vi "Variant to Meta Data.vi"(8 "Error In":errorcluster, 9 "Name":string, 11 "Value":variant) -> (0 "Error Out":errorcluster, 1 "Name out":string, 2 "deleted path":path, 3 "Meta data":string)   [LabVIEW 2016]
uses:
  <vilib>/Utility/config.llb/NI_LVConfig.lvlib
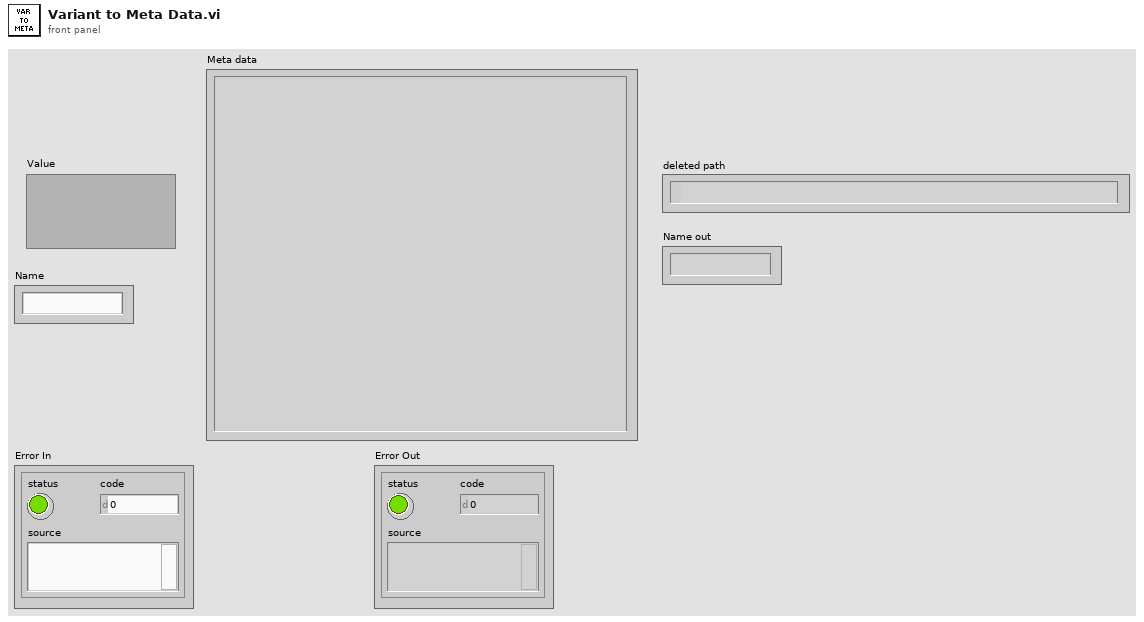
[diagram p1: front panel]
types:
  T1 = typedef "NI_LVConfig.lvlib/Config Data RefNum.ctl" = refnum<k1>
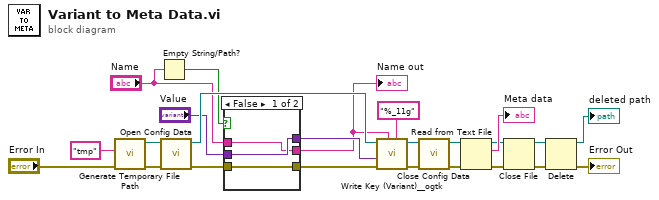
[diagram p0: block diagram]
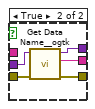
[diagram p2: hidden frame]
diagram:
  n1 = call <vilib>:"Generate Temporary File Path.vi"("error in (no error)"="Error In", "Temporary File Extension (tmp)"="tmp") -> ("error out"=w11:errorcluster, "Unique Temporary File Path"=w23:path)  [unwired: 8 in]
  n2 = Empty String/Path?(string/path="Name") -> (empty?=w7:bool)
  n3 = call <vilib>:"Open Config Data.vi"("error in (no error)"=w11, "configuration file path"=w23) -> ("error out"=w6:errorcluster, "refnum"=w22:T1)  [unwired: 7 in, 1 out]
  n4 = case shown="False" w7 {
    tunnel: "Value" -> [w27 w32]
    tunnel: [w25 w31] -> w2
    tunnel: w6 -> [w26 w30]
    tunnel: [w26 w29] -> w5
    tunnel: [w27 w28] -> w4
    tunnel: "Name" -> [w25 _]
    frame False {
    }
    frame True {
      n5 = call <userlib>:"Get Data Name__ogtk.vi"("error in (no error)"=w30, "Data"=w32) -> ("error out"=w29:errorcluster, "Data Name"=w31:string, "Data dup"=w28:variant)  [unwired: 7 in]
    }
  }
  "Name out" <- w2
  n6 = call <userlib>:"Write Key (Variant)__ogtk.vi"("float number format"="%_11g", "section"=w2, "error in (no error)"=w5, "key-value"=w4, "refnum"=w22) -> ("error out"=w21:errorcluster, "refnum out"=w20:T1)  [unwired: 5 in]
  n7 = call <vilib>:"Close Config Data.vi"("error in (no error)"=w21, "refnum"=w20) -> ("error out"=w18:errorcluster, "file path"=w19:path)  [unwired: 8 in]
  n8 = Read from Text File(file (use dialog)=w19, error in=w18) -> (refnum out=w16:refnum<file>, text=→"Meta data":string, error out=w15:errorcluster)  [unwired: 2 in, 1 out]
  n9 = Close File(refnum=w16, error in=w15) -> (path=w13:path, error out=w14:errorcluster)
  n10 = Delete(path (use dialog)=w13, error in=w14) -> (deleted path=→"deleted path":path, error out=→"Error Out":errorcluster)  [unwired: 3 in, 1 out]
